vi "Add.vi"(8 "error in":errorcluster, 10 "Sub Object":refnum<class "Sub Object.lvclass">, 11 "Sub Objects Dictionary in":refnum<class "Sub Objects Dictionary.lvclass">) -> (0 "error out":errorcluster, 3 "Sub Objects Dictionary out":refnum<class "Sub Objects Dictionary.lvclass">)   [LabVIEW 2020, in "CANopen.lvlib" / "Sub Objects Dictionary.lvclass"]
doc: "Adds an entry with the specified key and value into the Ordered Dictionary collection with the lowest available index."
uses:
  Sub Objects Dictionary.lvclass
  Sub Objects Dictionary.lvclass/Sub Objects Dictionary.ctl
  Sub Object/Sub Object.lvclass
  Ordered-Dictionary/Ordered Object Dictionary/Source/Ordered Object Dictionary.lvclass
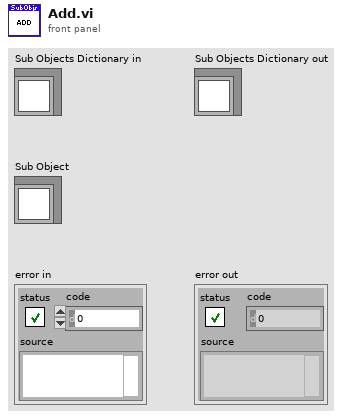
[diagram p1: front panel]
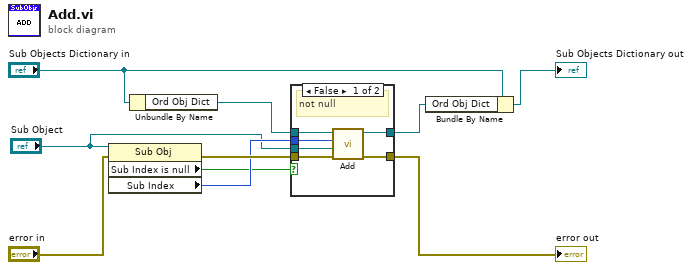
[diagram p0: block diagram]
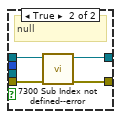
[diagram p2: hidden frame]
diagram:
  n1 = property class="Sub Obj"(reference="Sub Object", error in="error in") -> (error out=w8:errorcluster, "Sub Index is null"=w2:bool, "Sub Index"=w3:u8)  [unwired: 1 out]
  n2 = Unbundle By Name("Sub Objects Dictionary in") -> ("Ord Obj Dict"=w10:refnum<class "Ordered Object Dictionary.lvclass">)
  n3 = case shown="False" w2 {
    tunnel: w10 -> [w16 w19]
    tunnel: w8 -> [w15 w18]
    tunnel: [w14 w17] -> w7
    tunnel: [w13 w19] -> w4
    tunnel: w3 -> [w12 _]
    tunnel: "Sub Object" -> [w11 _]
    frame False {
      # "not null"
      n4 = call "Add.vi"("error in"=w15, "Value"=w11, "Key"=w12, "Ordered Object Dictionary in"=w16) -> ("error out"=w14:errorcluster, "Ordered Object Dictionary out"=w13:refnum<class "Ordered Object Dictionary.lvclass">)  [unwired: 6 in]
    }
    frame True {
      # "null"
      n5 = call "7300 Sub Index not defined--error.vi"("error in"=w18) -> ("error out"=w17:errorcluster)  [unwired: 9 in, 1 out]
    }
  }
  "error out" <- w7
  n6 = Bundle By Name(cluster="Sub Objects Dictionary in", "Ord Obj Dict"=w4) -> (→"Sub Objects Dictionary out":refnum<class "Sub Objects Dictionary.lvclass">)
